vi "Snap to bottom-left.vi"(1 "Fixed Rect":T1, 2 "Rect":T1) -> (0 "Snapped to bottom left":T1)   [LabVIEW 2012]
doc: "This VI calculates the position of a snapped-to-bottomleft rectangle from the positions of a fixed rectangle and a smaller one that will be positioned inside."
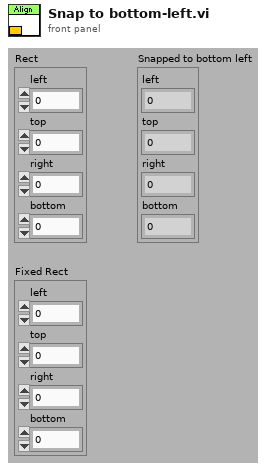
[diagram p1: front panel]
types:
  T1 = cluster{"left":i16, "top":i16, "right":i16, "bottom":i16}
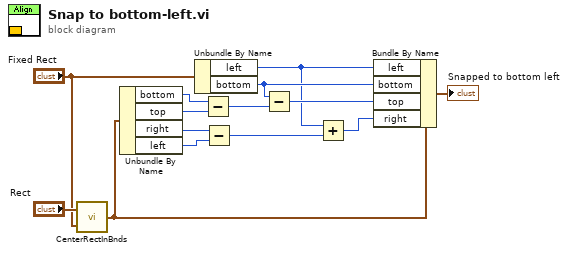
[diagram p0: block diagram]
diagram:
  n1 = call <vilib>:"CenterRectInBnds.vi"("bounds"="Fixed Rect", "rect"="Rect") -> ("centered rect"=w11:T1)
  n2 = Unbundle By Name(w11) -> ("bottom"=w14:i16, "top"=w13:i16, "right"=w5:i16, "left"=w4:i16)
  n3 = Unbundle By Name("Fixed Rect") -> ("left"=w3:i16, "bottom"=w9:i16)
  n4 = Subtract(x=w14, y=w13) -> (x-y=w12:i16)
  n5 = Subtract(x=w5, y=w4) -> (x-y=w2:i16)
  n6 = Subtract(x=w9, y=w12) -> (x-y=w10:i16)
  n7 = Add(x=w3, y=w2) -> (x+y=w1:i16)
  n8 = Bundle By Name(cluster=w11, "left"=w3, "bottom"=w9, "top"=w10, "right"=w1) -> (→"Snapped to bottom left":T1)
